vi "Initialization VI.vi"(8 "error in (no error)":errorcluster, 10 "Custom XML":string, 11 "Device Item Ref in":T1 format="%.0x") -> (0 "error out":errorcluster, 3 "Device Item Ref out":T1 format="%.0x")   [LabVIEW 2025, in "Runtime Configuration Support Inline Async Example System Explorer.lvlib"]
uses:
  <vilib>/NI VeriStand/Custom Device API/Custom Device Item Ref.ctl
  Runtime Configuration Support Inline Async Example System Explorer.lvlib
  <vilib>/NI VeriStand/Custom Device API/Set Item Property (U16).vi
  <vilib>/NI/NI VeriStand Custom Device Import and Export Tool/ImportExport.lvlib
  <vilib>/NI VeriStand/Custom Device API/Custom Device API.lvlib
  <vilib>/NI VeriStand/Custom Device API/Custom Device Channel Type.ctl
  <vilib>/NI VeriStand/Custom Device API/Custom Device Channel.ctl
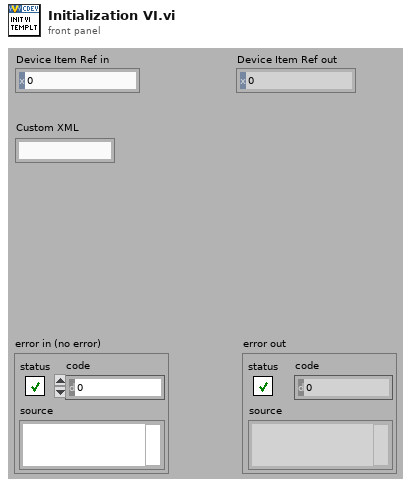
[diagram p1: front panel]
types:
  T1 = typedef "Custom Device API.lvlib/Custom Device Item Ref.ctl" = u64
  T2 = typedef "Custom Device API.lvlib/Custom Device Channel.ctl" = cluster{"Type":T3, "Units":string, "Default Value":dbl, "Faultable":bool, "Scalable":bool}
  T3 = typedef "Custom Device API.lvlib/Custom Device Channel Type.ctl" = enum16{"Input", "Output"}
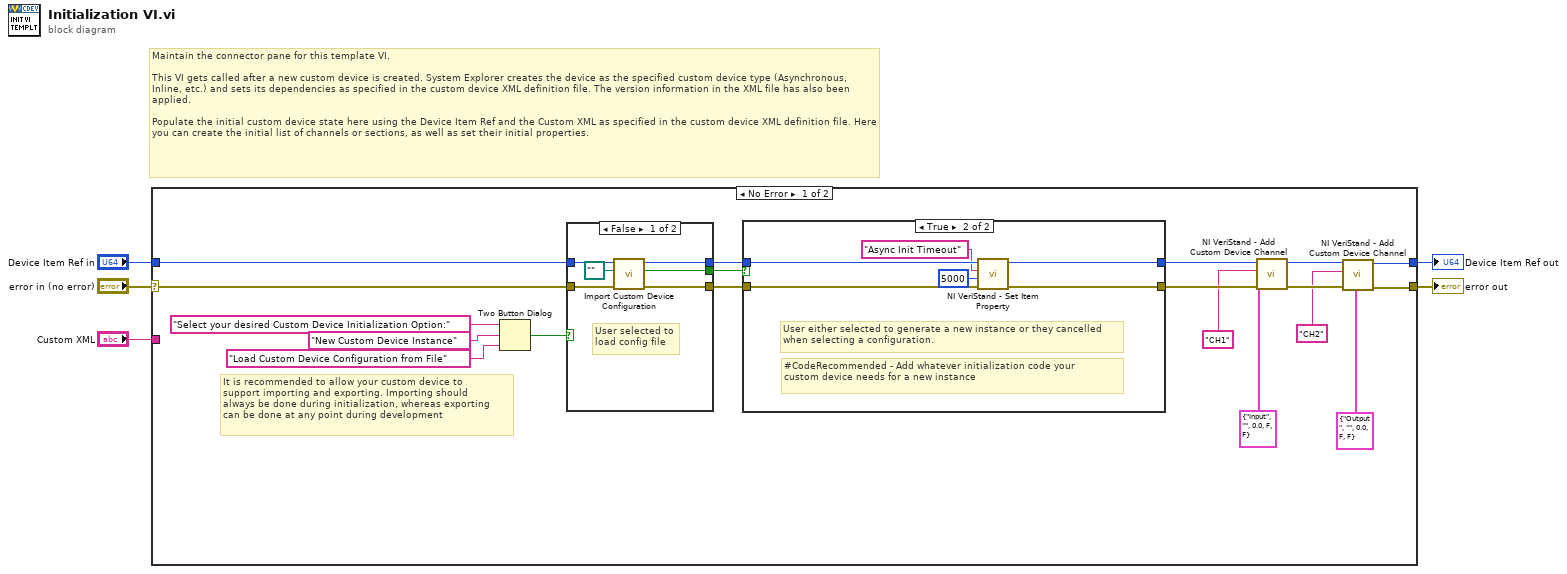
[diagram p0: block diagram]
diagram:
  # "Maintain the connector pane for this template VI.\n\nThis VI gets called after a new custom device is created. System Explorer creates the device as the specified custom device type (Asynchronous, Inline, etc.) and sets its dependencies as specified in the custom device XML definition file. The version information in the XML file has also been applied.\n\nPopulate the initial custom device state here using the Device Item Ref and the Custom XML as specified in the custom device XML definition file. Here you can create the initial list of channels or sections, as well as set their initial properties."
  n1 = case shown="No Error" "error in (no error)" {
    selector: "error in (no error)" -> [w19 w43]
    tunnel: [w8 w43] -> w5
    tunnel: [w10 w42] -> w3
    tunnel: "Device Item Ref in" -> [w20 w42]
    tunnel: "Custom XML" -> [_ _]
    frame No Error {
      # "It is recommended to allow your custom device to\nsupport importing and exporting. Importing should\nalways be done during initialization, whereas exporting\ncan be done at any point during development"
      n2 = Two Button Dialog(message="Select your desired Custom Device Initialization Option:", 1:"Load Custom Device Configuration from File" ("F button name (\"Cancel\")"), 2:"New Custom Device Instance" ("T button name (\"OK\")")) -> (T button?=w21:bool)
      n3 = case "New or Load" shown="False" w21 {
        selector: w21 -> [_ w39]
        tunnel: w20 -> [w38 w41]
        tunnel: [w37 w41] -> w18
        tunnel: w19 -> [w35 w40]
        tunnel: [w34 w40] -> w16
        tunnel: [w33 w39] -> w17
        frame False {
          # "User selected to\nload config file"
          n4 = call <vilib>:"Import Custom Device Configuration.vi"("error in (no error)"=w35, "Path"=path "", "NodeID"=w38) -> ("error out"=w34:errorcluster, "cancelled"=w33:bool, "NodeID out"=w37:u64)  [unwired: 6 in]
        }
        frame True {
          # "User selected new\ncustom device. Do\nnothing in this case\nand handle new\ngeneration in the\nnext case structure"
        }
      }
      n5 = case "Create New" shown="True" w17 {
        tunnel: w18 -> [w26 w30]
        tunnel: w16 -> [w25 w31]
        tunnel: [w25 w29] -> w15
        tunnel: [w26 w28] -> w14
        frame False {
          # "User selected to import from configuration and didn't cancel import"
        }
        frame True {
          # "#CodeRecommended - Add whatever initialization code your\ncustom device needs for a new instance"
          # "User either selected to generate a new instance or they cancelled\nwhen selecting a configuration."
          n6 = call-poly <vilib>:"NI VeriStand - Set Item Property.vi"("error in (no error)"=w31, "Value"=u16 5000, "Property Name"="Async Init Timeout", "Item Ref in"=w30) -> ("error out"=w29:errorcluster, "Item Ref out"=w28:T1)  [unwired: 5 in, 1 out]
        }
      }
      n7 = call <vilib>:"NI VeriStand - Add Custom Device Channel.vi"("error in (no error)"=w15, "Channel"=T2 {"Type"=enum."Input", "Units"="", "Default Value"=0.0, "Faultable"=FALSE, "Scalable"=FALSE}, "Channel Name"="CH1", "Parent Ref in"=w14) -> ("error out"=w9:errorcluster, "Parent Ref out"=w11:T1)  [unwired: 4 in, 2 out]
      n8 = call <vilib>:"NI VeriStand - Add Custom Device Channel.vi"("error in (no error)"=w9, "Channel"=T2 {"Type"=enum."Output", "Units"="", "Default Value"=0.0, "Faultable"=FALSE, "Scalable"=FALSE}, "Channel Name"="CH2", "Parent Ref in"=w11) -> ("error out"=w8:errorcluster, "Parent Ref out"=w10:T1)  [unwired: 4 in, 2 out]
    }
    frame Error {
    }
  }
  "error out" <- w5
  "Device Item Ref out" <- w3
